vi "实时小时数据单参数上传.vi"(0 "参数数值":T1={"CODMn"=TRUE, "CODCr"=TRUE, "DO"=TRUE, "铜"=TRUE, "PH"=TRUE, "氨氮"=TRUE, "比电导率"=TRUE, "水温"=TRUE, "COD"=TRUE, "浊度"=TRUE, "总氮"=TRUE, "总磷"=TRUE, "叶绿素a"=TRUE, "藻密度"=TRUE, "水位"=TRUE, "流速"=TRUE, "瞬时流量"=TRUE, "累积流量"=TRUE, "亚硝氮"=TRUE, "硫化物"=TRUE, "ORP"=TRUE, "铅"=TRUE, "镉"=TRUE, "锌"=TRUE, "镍"=TRUE, "锰"=TRUE, "汞"=TRUE}) -> (4 "数据发送起始时间":timestamp format="%<%.3X\n%Y/%m/%d>T", 15 "error out":errorcluster)   [LabVIEW 2016, in "数据传输系统.lvlib"]
uses:
  <vilib>/Utility/config.llb/Write Key (String).vi
  <vilib>/Utility/config.llb/NI_LVConfig.lvlib
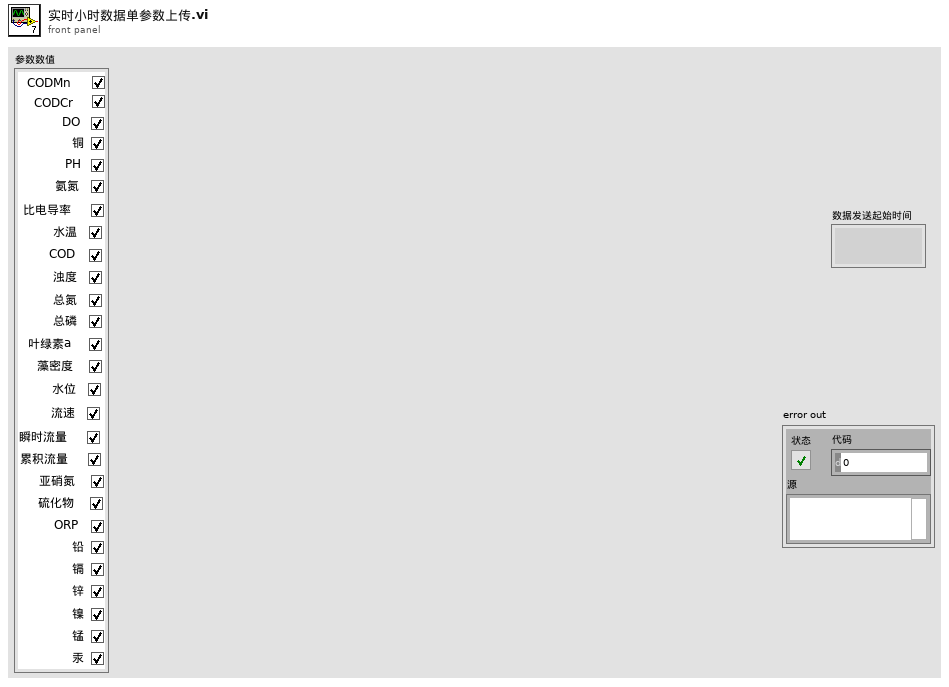
[diagram p1: front panel]
types:
  T1 = cluster{"CODMn":bool, "CODCr":bool, "DO":bool, "铜":bool, "PH":bool, "氨氮":bool, "比电导率":bool, "水温":bool, "COD":bool, "浊度":bool, "总氮":bool, "总磷":bool, "叶绿素a":bool, "藻密度":bool, "水位":bool, "流速":bool, "瞬时流量":bool, "累积流量":bool, "亚硝氮":bool, "硫化物":bool, "ORP":bool, "铅":bool, "镉":bool, "锌":bool, "镍":bool, "锰":bool, "汞":bool}
  T2 = cluster{"CODMn":bool, "CODCr":bool, "DO":bool, "铜":bool, "PH":bool, "氨氮":bool, "比电导率":bool, "水温":bool, "COD":bool, "浊度":bool, "总氮":bool, "总磷":bool, "叶绿素a":bool, "藻密度":bool, "水位":bool, "流速":bool, "瞬时流量":bool, "累积流量":bool, "亚硝酸盐":bool, "硫化物":bool, "ORP":bool, "铅":bool, "镉":bool, "锌":bool, "镍":bool, "锰":bool, "汞":bool}
  T3 = cluster{"time1":string, "time2":string, "time3":string, "time4":string, "time5":string, "time6":string, "time7":string, "time8":string, "time9":string, "time10":string, "time11":string, "time12":string, "time13":string, "time14":string, "time15":string, "time16":string, "time17":string, "time18":string, "time19":string, "time20":string, "time21":string, "time22":string, "time23":string, "time24":string, "time25":string, "time26":string, "time27":string}
  T4 = typedef "NI_LVConfig.lvlib/Config Data RefNum.ctl" = refnum<k1>
  T5 = cluster{"水样数据索引[0]":string, "水样数据索引[1]":string, "水样数据索引[2]":string, "水样数据索引[3]":string, "水样数据索引[4]":string, "水样数据索引[5]":string, "水样数据索引[6]":string, "水样数据索引[7]":string, "水样数据索引[8]":string, "水样数据索引[9]":string, "水样数据索引[10]":string, "水样数据索引[11]":string, "水样数据索引[12]":string, "水样数据索引[13]":string, "水样数据索引[14]":string, "水样数据索引[15]":string, "水样数据索引[16]":string, "水样数据索引[17]":string, "水样数据索引[18]":string, "水样数据索引[19]":string, "水样数据索引[20]":string, "水样数据索引[21]":string, "水样数据索引[22]":string, "水样数据索引[23]":string, "水样数据索引[24]":string, "水样数据索引[25]":string, "水样数据索引[26]":string}
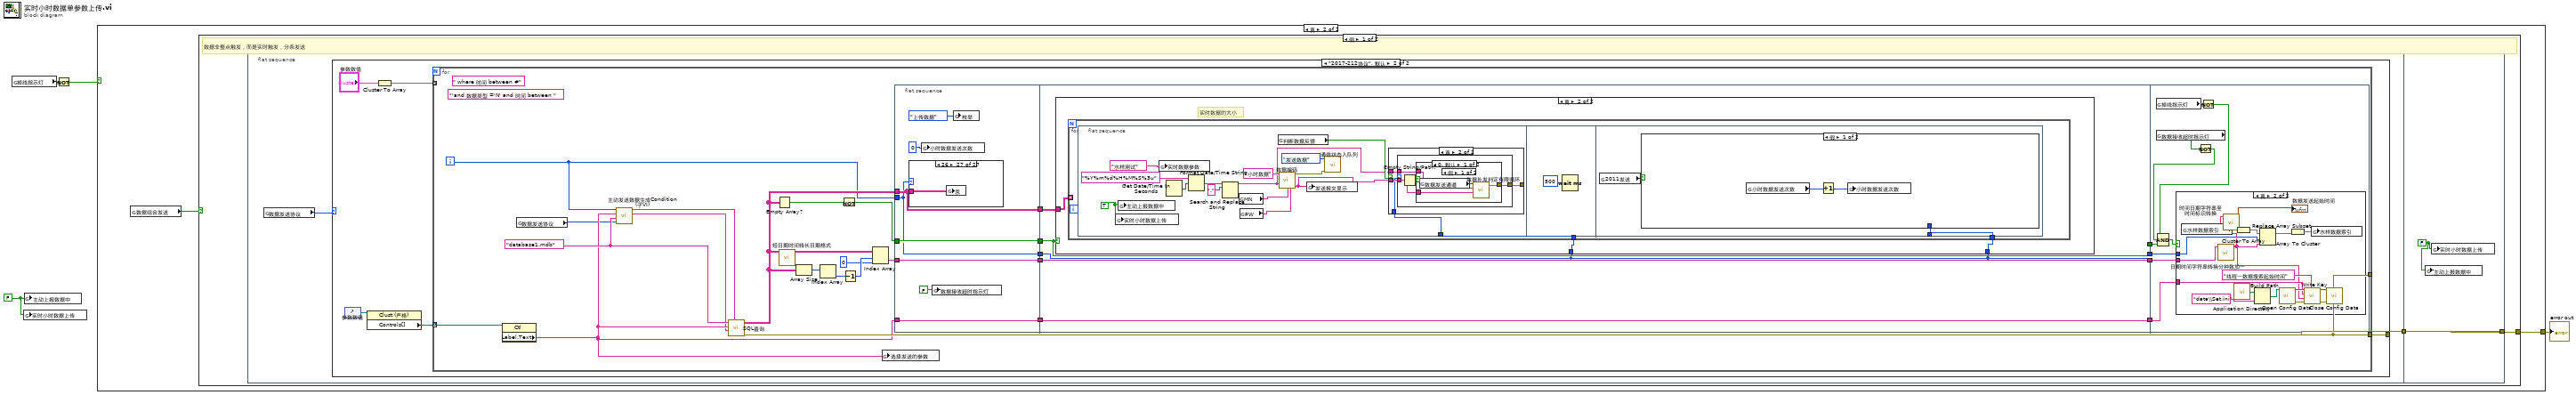
[diagram p0: block diagram]
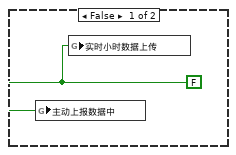
[diagram p2: hidden frame]
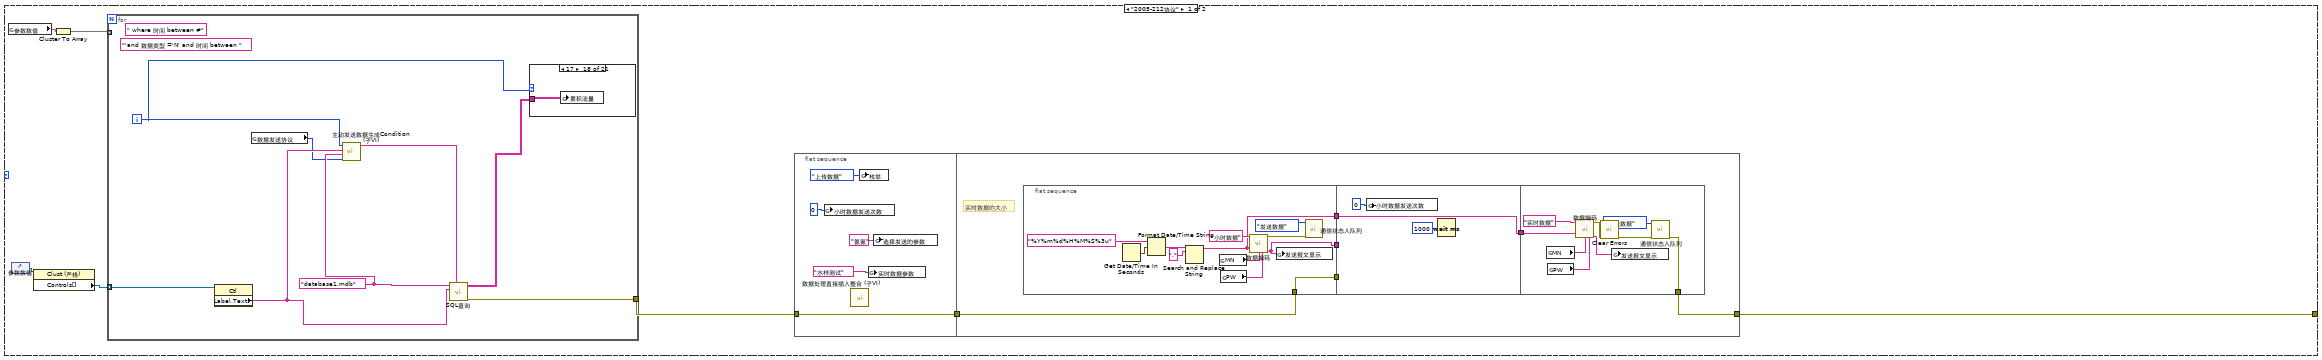
[diagram p3: hidden frame]
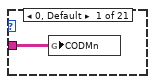
[diagram p4: hidden frame]
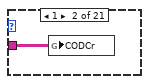
[diagram p5: hidden frame]
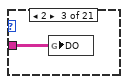
[diagram p6: hidden frame]
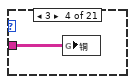
[diagram p7: hidden frame]
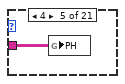
[diagram p8: hidden frame]
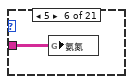
[diagram p9: hidden frame]
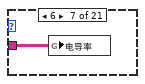
[diagram p10: hidden frame]
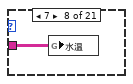
[diagram p11: hidden frame]
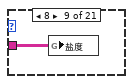
[diagram p12: hidden frame]
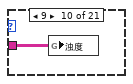
[diagram p13: hidden frame]
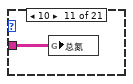
[diagram p14: hidden frame]
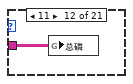
[diagram p15: hidden frame]
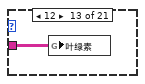
[diagram p16: hidden frame]
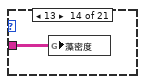
[diagram p17: hidden frame]
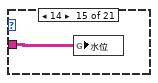
[diagram p18: hidden frame]
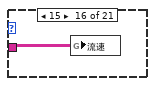
[diagram p19: hidden frame]
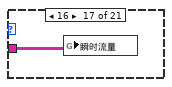
[diagram p20: hidden frame]
diagram:
  w1 = FALSE ("小时数据上传")
  n1 = global read "全局 数据发送重叠.vi" "掉线指示灯"() -> (w4:bool)
  n2 = global write "全局1.vi" "实时小时数据上传"(w1) -> ()
  n3 = global write "全局 数据发送重叠.vi" "主动上报数据中"(w1) -> ()
  n4 = Not(x=w4) -> (.not. x?=w3:bool)
  n5 = case shown="真" w3 {
    tunnel: [_ w7] -> w2
    frame False {
      w5 = FALSE ("小时数据上传")
      n6 = global write "全局 数据发送重叠.vi" "主动上报数据中"(w5) -> ()
      n7 = global write "全局1.vi" "实时小时数据上传"(w5) -> ()
    }
    frame True {
      n8 = global read "断电保存全局.vi" "数据组合发送"() -> (w6:bool)
      n9 = case shown="假" w6 {
        tunnel: [w8 _] -> w7
        frame False {
          # "数据非整点触发，而是实时触发，分条发送"
          n10 = flat-sequence {
            tunnel: [w11] -> w9
            tunnel: [w241] -> w8
            tunnel: w9 -> [w241]
            frame #0 {
              n11 = global read "断电保存全局.vi" "数据发送协议"() -> (w10:enum16{"2005-212协议", "2017-212协议"})
              n12 = case shown="\"2017-212协议\", 默认" w10 {
                tunnel: [w12 w86] -> w11
                frame "2005-212协议" {
                  n13 = global read "全局1.vi" "参数数值"() -> (w15:T2)
                  n14 = control-ref of="参数数值"() -> (w14:refnum<vi>)
                  n15 = property class="Clust (严格)"(reference=w14) -> ("Controls[]"=w13:refnum<vi>[])  [unwired: 1 in, 2 out]
                  n16 = Cluster To Array(cluster=w15) -> (array=w18:bool[])
                  n17 = for {
                    tunnel: w18 -> [_] mode=indexing
                    tunnel: [w61] -> w17
                    tunnel: w13 -> [w56] mode=indexing
                    i -> [w54]
                    (unwired) " where 时间 between #"
                    w59 = "database1.mdb" ("database")
                    (unwired) "'and 数据类型 ='N' and 时间 between "
                    n18 = property class="Ctl"(reference=w56) -> ("Label.Text"=w60:string)  [unwired: 1 in, 2 out]
                    n19 = global read "断电保存全局.vi" "数据发送协议"() -> (w57:enum16{"2005-212协议", "2017-212协议"})
                    n20 = call "主动发送数据生成Condition(子VI).vi"("数据发送协议"=w57, "database"=w59, "Label.Text"=w60, "数值"=w54) -> ("CONDITION"=w58:string)  [unwired: 6 in, 1 out]
                    n21 = call "SQL查询.vi"("condition"=w58, "table输入"=w60, "database"=w59) -> ("error out"=w61:errorcluster, "data"=w55:string[][])  [unwired: 6 in, 1 out]
                    n22 = case shown="17" w54 {
                      tunnel: w55 -> [w62 w63 w64 w65 w66 w67 w68 w69 w70 w71 w72 w73 w74 w75 w76 w77 w78 w79 w80 w81 w82]
                      frame 0, Default {
                        n23 = global write "全局 所有参数.vi" "CODMn"(w62) -> ()
                      }
                      frame 1 {
                        n24 = global write "全局 所有参数.vi" "CODCr"(w63) -> ()
                      }
                      frame 2 {
                        n25 = global write "全局 所有参数.vi" "DO"(w64) -> ()
                      }
                      frame 3 {
                        n26 = global write "全局 所有参数.vi" "铜"(w65) -> ()
                      }
                      frame 4 {
                        n27 = global write "全局 所有参数.vi" "PH"(w66) -> ()
                      }
                      frame 5 {
                        n28 = global write "全局 所有参数.vi" "氨氮"(w67) -> ()
                      }
                      frame 6 {
                        n29 = global write "全局 所有参数.vi" "电导率"(w68) -> ()
                      }
                      frame 7 {
                        n30 = global write "全局 所有参数.vi" "水温"(w69) -> ()
                      }
                      frame 8 {
                        n31 = global write "全局 所有参数.vi" "盐度"(w70) -> ()
                      }
                      frame 9 {
                        n32 = global write "全局 所有参数.vi" "浊度"(w71) -> ()
                      }
                      frame 10 {
                        n33 = global write "全局 所有参数.vi" "总氮"(w72) -> ()
                      }
                      frame 11 {
                        n34 = global write "全局 所有参数.vi" "总磷"(w73) -> ()
                      }
                      frame 12 {
                        n35 = global write "全局 所有参数.vi" "叶绿素"(w74) -> ()
                      }
                      frame 13 {
                        n36 = global write "全局 所有参数.vi" "藻密度"(w75) -> ()
                      }
                      frame 14 {
                        n37 = global write "全局 所有参数.vi" "水位"(w76) -> ()
                      }
                      frame 15 {
                        n38 = global write "全局 所有参数.vi" "流速"(w77) -> ()
                      }
                      frame 16 {
                        n39 = global write "全局 所有参数.vi" "瞬时流量"(w78) -> ()
                      }
                      frame 17 {
                        n40 = global write "全局 所有参数.vi" "累积流量"(w79) -> ()
                      }
                      frame 18 {
                        n41 = global write "全局 所有参数.vi" "亚硝酸盐"(w80) -> ()
                      }
                      frame 19 {
                        n42 = global write "全局 所有参数.vi" "硫化物"(w81) -> ()
                      }
                      frame 20 {
                        n43 = global write "全局 所有参数.vi" "ORP"(w82) -> ()
                      }
                    }
                  }
                  n44 = flat-sequence {
                    tunnel: w17 -> [w19]
                    tunnel: [w19] -> w16
                    tunnel: w16 -> [w27]
                    tunnel: [w26] -> w12
                    frame #0 {
                      n45 = global write "全局 小时数据发送次数.vi" "小时数据发送次数"(0 ("小时数据发送次数")) -> ()
                      n46 = call "数据处理直接插入整合 (子VI).vi"() -> ()  [unwired: 12 in]
                      n47 = global write "全局1.vi" "枚举"(enum16{"返回请求应答", "上传数据", "返回执行结果"}."上传数据" ("枚举")) -> ()
                      n48 = global write "全局 实时数据参数.vi" "实时数据参数"("水样测试" ("实时数据参数")) -> ()
                      n49 = global write "全局 水样时间.vi" "选择发送的参数"("氨氮" ("选择发送的参数")) -> ()
                    }
                    frame #1 {
                      # "实时数据的大小"
                      n50 = flat-sequence {
                        tunnel: [w36] -> w29
                        tunnel: [w31] -> w28
                        tunnel: w27 -> [w31]
                        tunnel: [w30] -> w25
                        tunnel: w29 -> [_]
                        tunnel: w28 -> [_]
                        tunnel: w25 -> [w42]
                        tunnel: [w42] -> w24
                        tunnel: [w47] -> w26
                        tunnel: w24 -> [w46]
                        frame #0 {
                          n51 = Get Date/Time In Seconds() -> (seconds since 1Jan1904=w39:timestamp)
                          n52 = Format Date/Time String(time format string (%c)="%Y%m%d%H%M%S%3u" ("时间格式字符串(%c)"), seconds (now)=w39) -> (date/time string=w40:string)  [unwired: 1 in]
                          n53 = Search and Replace String(input string=w40, search string="." ("搜索字符串")) -> (result string=w30:string)  [unwired: 6 in, 3 out]
                          n54 = global read "断电保存全局.vi" "MN"() -> (w34:string)
                          n55 = global read "断电保存全局.vi" "PW"() -> (w33:string)
                          n56 = call "数据编码.vi"("table输入"="小时数据" ("新元素/子数组"), "QN"=w30, "MN"=w34, "PW"=w33) -> ("错误常量"=w32:errorcluster, "通讯包字符串"=w36:string)  [unwired: 10 in]
                          n57 = global write "全局1.vi" "发送报文显示"(w36) -> ()
                          n58 = call "通信状态入队列.vi"("错误输入（无错误）"=w32, "枚举"=enum16{"打开连接", "发送数据", "读取数据", "数据处理", "关闭连接"}."发送数据") -> ()  [unwired: 9 in, 1 out]
                        }
                        frame #1 {
                          n59 = global write "全局 小时数据发送次数.vi" "小时数据发送次数"(0 ("小时数据发送次数")) -> ()
                          n60 = Wait (ms)(milliseconds to wait=u32 1000 ("等待时间（毫秒）")) -> ()  [unwired: 1 out]
                        }
                        frame #2 {
                          n61 = global read "断电保存全局.vi" "MN"() -> (w49:string)
                          n62 = global read "断电保存全局.vi" "PW"() -> (w50:string)
                          n63 = call "数据编码.vi"("table输入"="实时数据" ("新元素/子数组"), "QN"=w46, "MN"=w49, "PW"=w50) -> ("错误常量"=w48:errorcluster, "通讯包字符串"=w52:string)  [unwired: 10 in]
                          n64 = call <vilib>:"Clear Errors.vi"("error in (no error)"=w48) -> ("error out"=w45:errorcluster)  [unwired: 5 in, 1 out]
                          n65 = global write "全局1.vi" "发送报文显示"(w52) -> ()
                          n66 = call "通信状态入队列.vi"("错误输入（无错误）"=w45, "枚举"=enum16{"打开连接", "发送数据", "读取数据", "数据处理", "关闭连接"}."发送数据") -> ("错误输出"=w47:errorcluster)  [unwired: 9 in]
                        }
                      }
                    }
                  }
                }
                frame "2017-212协议", Default {
                  n67 = control-ref of="参数数值"() -> (w85:refnum<vi>)
                  n68 = property class="Clust (严格)"(reference=w85) -> ("Controls[]"=w84:refnum<vi>[])  [unwired: 1 in, 2 out]
                  n69 = Cluster To Array(cluster="参数数值") -> (array=w87:bool[])
                  n70 = for {
                    tunnel: w87 -> [_] mode=indexing
                    tunnel: [w99] -> w86
                    tunnel: [w99] -> _
                    tunnel: w84 -> [w89] mode=indexing
                    i -> [w90]
                    (unwired) " where 时间 between #"
                    w98 = "database1.mdb" ("database")
                    (unwired) "'and 数据类型 ='N' and 时间 between "
                    n71 = property class="Ctl"(reference=w89) -> ("Label.Text"=w97:string)  [unwired: 1 in, 2 out]
                    n72 = global read "断电保存全局.vi" "数据发送协议"() -> (w96:enum16{"2005-212协议", "2017-212协议"})
                    n73 = call "主动发送数据生成Condition(子VI).vi"("数据发送协议"=w96, "database"=w98, "Label.Text"=w97, "数值"=w90) -> ("columns"=w88:string[], "CONDITION"=w113:string)  [unwired: 6 in]
                    n74 = call "SQL查询.vi"("condition"=w113, "columns"=w88, "table输入"=w97, "database"=w98) -> ("error out"=w99:errorcluster, "data"=w93:string[][])  [unwired: 5 in, 1 out]
                    n75 = Empty Array?(array=w93) -> (empty?=w112:bool)
                    n76 = call "短日期时间转长日期格式.vi"("data"=w93) -> ("输出数组"=w111:string[][])  [unwired: 10 in]
                    n77 = Array Size(array=w93) -> (size(s)=w95:i32[])
                    n78 = Index Array(array=w95) -> (element=w94:i32)  [unwired: 1 in]
                    n79 = Not(x=w112) -> (.not. x?=w108:bool)
                    n80 = Decrement(x=w94) -> (x-1=w92:i32)
                    n81 = Index Array(array=w111, index (row)=w92, index (col)=0 ("禁用的索引 (列)")) -> (element=w105:string)
                    n82 = global write "全局 水样时间.vi" "选择发送的参数"(w97) -> ()
                    n83 = flat-sequence {
                      tunnel: [w121] -> w110
                      tunnel: [w120] -> w109
                      tunnel: w108 -> [w121]
                      tunnel: w93 -> [w120]
                      tunnel: w90 -> [w115]
                      tunnel: w97 -> [w117]
                      tunnel: [w117] -> w106
                      tunnel: w105 -> [w116]
                      tunnel: [w116] -> w103
                      tunnel: [w115] -> w100
                      tunnel: w110 -> [w150]
                      tunnel: w109 -> [w153]
                      tunnel: [w152] -> w107
                      tunnel: w106 -> [w152]
                      tunnel: [w151] -> w104
                      tunnel: w103 -> [w151]
                      tunnel: [w150] -> w102
                      tunnel: [w149] -> w101
                      tunnel: w100 -> [w149]
                      tunnel: w107 -> [w222]
                      tunnel: w104 -> [w221]
                      tunnel: w102 -> [w219]
                      tunnel: w101 -> [w220]
                      frame #0 {
                        n84 = case shown="26" w115 {
                          tunnel: w120 -> [w122 w123 w124 w125 w126 w127 w128 w129 w130 w131 w132 w133 w134 w135 w136 w137 w138 w139 w140 w141 w142 w143 w144 w145 w146 w147 w148]
                          frame 0, Default {
                            n85 = global write "全局 所有参数.vi" "CODMn"(w122) -> ()
                          }
                          frame 1 {
                            n86 = global write "全局 所有参数.vi" "CODCr"(w123) -> ()
                          }
                          frame 2 {
                            n87 = global write "全局 所有参数.vi" "DO"(w124) -> ()
                          }
                          frame 3 {
                            n88 = global write "全局 所有参数.vi" "铜"(w125) -> ()
                          }
                          frame 4 {
                            n89 = global write "全局 所有参数.vi" "PH"(w126) -> ()
                          }
                          frame 5 {
                            n90 = global write "全局 所有参数.vi" "氨氮"(w127) -> ()
                          }
                          frame 6 {
                            n91 = global write "全局 所有参数.vi" "电导率"(w128) -> ()
                          }
                          frame 7 {
                            n92 = global write "全局 所有参数.vi" "水温"(w129) -> ()
                          }
                          frame 8 {
                            n93 = global write "全局 所有参数.vi" "盐度"(w130) -> ()
                          }
                          frame 9 {
                            n94 = global write "全局 所有参数.vi" "浊度"(w131) -> ()
                          }
                          frame 10 {
                            n95 = global write "全局 所有参数.vi" "总氮"(w132) -> ()
                          }
                          frame 11 {
                            n96 = global write "全局 所有参数.vi" "总磷"(w133) -> ()
                          }
                          frame 12 {
                            n97 = global write "全局 所有参数.vi" "叶绿素"(w134) -> ()
                          }
                          frame 13 {
                            n98 = global write "全局 所有参数.vi" "藻密度"(w135) -> ()
                          }
                          frame 14 {
                            n99 = global write "全局 所有参数.vi" "水位"(w136) -> ()
                          }
                          frame 15 {
                            n100 = global write "全局 所有参数.vi" "流速"(w137) -> ()
                          }
                          frame 16 {
                            n101 = global write "全局 所有参数.vi" "瞬时流量"(w138) -> ()
                          }
                          frame 17 {
                            n102 = global write "全局 所有参数.vi" "累积流量"(w139) -> ()
                          }
                          frame 18 {
                            n103 = global write "全局 所有参数.vi" "亚硝酸盐"(w140) -> ()
                          }
                          frame 19 {
                            n104 = global write "全局 所有参数.vi" "硫化物"(w141) -> ()
                          }
                          frame 20 {
                            n105 = global write "全局 所有参数.vi" "ORP"(w142) -> ()
                          }
                          frame 21 {
                            n106 = global write "全局 所有参数.vi" "铅"(w143) -> ()
                          }
                          frame 22 {
                            n107 = global write "全局 所有参数.vi" "镉"(w144) -> ()
                          }
                          frame 23 {
                            n108 = global write "全局 所有参数.vi" "锌"(w145) -> ()
                          }
                          frame 24 {
                            n109 = global write "全局 所有参数.vi" "镍"(w146) -> ()
                          }
                          frame 25 {
                            n110 = global write "全局 所有参数.vi" "锰"(w147) -> ()
                          }
                          frame 26 {
                            n111 = global write "全局 所有参数.vi" "汞"(w148) -> ()
                          }
                        }
                        n112 = global write "全局 小时数据发送次数.vi" "小时数据发送次数"(0 ("小时数据发送次数")) -> ()
                        n113 = global write "全局 数据发送重叠.vi" "数据接收超时指示灯"(FALSE ("数据接收超时指示灯")) -> ()
                        n114 = global write "全局1.vi" "枚举"(enum16{"返回请求应答", "上传数据", "返回执行结果"}."上传数据" ("枚举")) -> ()
                      }
                      frame #1 {
                        n115 = case shown="真" w150 {
                          tunnel: w153 -> [_ w156]
                          tunnel: w149 -> [_ w155]
                          tunnel: w149 -> [_ w154]
                          frame False {
                          }
                          frame True {
                            # "实时数据的大小"
                            n116 = for {
                              tunnel: w156 -> [_] mode=indexing
                              tunnel: w155 -> [w158]
                              tunnel: w154 -> [w157]
                              n117 = flat-sequence {
                                tunnel: w158 -> [w173]
                                tunnel: w157 -> [w187]
                                frame #0 {
                                w160 = TRUE ("小时数据上传")
                                n118 = global write "全局1.vi" "实时小时数据上传"(w160) -> ()
                                n119 = global write "全局 数据发送重叠.vi" "主动上报数据中"(w160) -> ()
                                n120 = global write "全局 实时数据参数.vi" "实时数据参数"("水样测试" ("实时数据参数")) -> ()
                                n121 = Get Date/Time In Seconds() -> (seconds since 1Jan1904=w170:timestamp)
                                n122 = Format Date/Time String(time format string (%c)="%Y%m%d%H%M%S%3u" ("时间格式字符串(%c)"), seconds (now)=w170) -> (date/time string=w171:string)  [unwired: 1 in]
                                n123 = Search and Replace String(input string=w171, search string="." ("搜索字符串")) -> (result string=w159:string)  [unwired: 6 in, 3 out]
                                n124 = global read "断电保存全局.vi" "MN"() -> (w166:string)
                                n125 = global read "断电保存全局.vi" "PW"() -> (w165:string)
                                n126 = global read "断电保存全局.vi" "判断数据反馈"() -> (w162:bool)
                                n127 = call "数据编码.vi"("table输入"="小时数据" ("新元素/子数组"), "QN"=w159, "MN"=w166, "PW"=w165) -> ("错误常量"=w163:errorcluster, "通讯包字符串"=w161:string)  [unwired: 10 in]
                                n128 = global write "全局1.vi" "发送报文显示"(w161) -> ()
                                n129 = call "通信状态入队列.vi"("错误输入（无错误）"=w163, "枚举"=enum16{"打开连接", "发送数据", "读取数据", "数据处理", "关闭连接"}."发送数据") -> ()  [unwired: 9 in, 1 out]
                                n130 = case shown="真" w162 {
                                tunnel: [_ w177] -> _
                                tunnel: w161 -> [_ w176]
                                tunnel: w173 -> [_ w175]
                                tunnel: w159 -> [_ w174]
                                frame False {
                                }
                                frame True {
                                n131 = case shown="0, 默认" w175 {
                                tunnel: [w180 _] -> w177
                                tunnel: w176 -> [w179 _]
                                tunnel: w174 -> [w178 _]
                                frame 0, Default {
                                n132 = Empty String/Path?(string/path=w179) -> (empty?=w181:bool)
                                n133 = case shown="假" w181 {
                                tunnel: [w185 _] -> w180
                                tunnel: w179 -> [w184 _]
                                tunnel: w178 -> [w182 _]
                                frame False {
                                n134 = global read "断电保存全局.vi" "数据发送通道"() -> (w183:enum16{"TCP", "VISA"})
                                n135 = call "数据补发判定有限循环.vi"("数据输入"=w184, "QN"=w182, "数据发送通道"=w183) -> ("error out"=w185:errorcluster)  [unwired: 8 in]
                                }
                                frame True {
                                }
                                }
                                }
                                frame 14..17 {
                                }
                                }
                                }
                                }
                                }
                                frame #1 {
                                n136 = Wait (ms)(milliseconds to wait=u32 500 ("等待时间（毫秒）")) -> ()  [unwired: 1 out]
                                }
                                frame #2 {
                                n137 = global read "断电保存全局.vi" "2011发送"() -> (w188:bool)
                                n138 = case shown="假" w188 {
                                tunnel: w187 -> [_ w205]
                                frame False {
                                n139 = global read "全局 小时数据发送次数.vi" "小时数据发送次数"() -> (w190:i32)
                                n140 = Increment(x=w190) -> (x+1=w189:i32)
                                n141 = global write "全局 小时数据发送次数.vi" "小时数据发送次数"(w189) -> ()
                                }
                                frame True {
                                n142 = Get Date/Time In Seconds() -> (seconds since 1Jan1904=w193:timestamp)
                                n143 = Format Date/Time String(time format string (%c)="%Y%m%d%H%M%S%3u" ("时间格式字符串(%c)"), seconds (now)=w193) -> (date/time string=w194:string)  [unwired: 1 in]
                                n144 = global read "断电保存全局.vi" "MN"() -> (w200:string)
                                n145 = global read "断电保存全局.vi" "PW"() -> (w199:string)
                                n146 = Search and Replace String(input string=w194, search string="." ("搜索字符串")) -> (result string=w191:string)  [unwired: 6 in, 3 out]
                                n147 = global write "全局 实时数据参数.vi" "实时数据参数"("水样测试" ("实时数据参数")) -> ()
                                n148 = call "数据编码.vi"("table输入"="实时数据" ("新元素/子数组"), "QN"=w191, "MN"=w200, "PW"=w199) -> ("错误常量"=w201:errorcluster, "通讯包字符串"=w196:string)  [unwired: 10 in]
                                n149 = global write "全局1.vi" "发送报文显示"(w196) -> ()
                                n150 = call "通信状态入队列.vi"("错误输入（无错误）"=w201, "枚举"=enum16{"打开连接", "发送数据", "读取数据", "数据处理", "关闭连接"}."发送数据") -> ("错误输出"=w198:errorcluster)  [unwired: 9 in]
                                n151 = global read "断电保存全局.vi" "判断数据反馈"() -> (w197:bool)
                                n152 = case shown="真" w197 {
                                tunnel: w196 -> [_ w209]
                                tunnel: w198 -> [_ w208]
                                tunnel: w205 -> [_ w207]
                                tunnel: w191 -> [_ w206]
                                frame False {
                                }
                                frame True {
                                n153 = case shown="0, 默认" w207 {
                                tunnel: w209 -> [w213 _]
                                tunnel: w208 -> [w212 _]
                                tunnel: w206 -> [w210 _]
                                frame 0, Default {
                                n154 = global read "断电保存全局.vi" "数据发送通道"() -> (w211:enum16{"TCP", "VISA"})
                                n155 = call "数据补发判定有限循环.vi"("错误输入（无错误）"=w212, "数据输入"=w213, "QN"=w210, "数据发送通道"=w211) -> ()  [unwired: 7 in, 1 out]
                                }
                                frame 14..17 {
                                }
                                }
                                }
                                }
                                }
                                }
                                }
                              }
                            }
                          }
                        }
                      }
                      frame #2 {
                        n156 = global read "全局 数据发送重叠.vi" "掉线指示灯"() -> (w215:bool)
                        n157 = global read "全局 数据发送重叠.vi" "数据接收超时指示灯"() -> (w216:bool)
                        n158 = Not(x=w216) -> (.not. x?=w217:bool)
                        n159 = Not(x=w215) -> (.not. x?=w214:bool)
                        n160 = Compound Arithmetic op=AND ("复合运算")(w214, w217, w219) -> (w218:bool)
                        n161 = case shown="真" w218 {
                          tunnel: w221 -> [_ w230]
                          tunnel: w220 -> [_ w224]
                          tunnel: w222 -> [_ w231]
                          frame False {
                          }
                          frame True {
                            n162 = global read "全局 水样时间.vi" "水样数据索引"() -> (w225:T3)
                            n163 = call "日期时间字符串转换分钟数加一.vi"("data[0]"=w230) -> ("日期/时间字符串"=w223:string)  [unwired: 10 in]
                            n164 = call "时间日期字符串至时间标识转换.vi"("时间日期字符串"=w223) -> ("时间标识"=→"数据发送起始时间":timestamp)  [unwired: 10 in]
                            n165 = call <vilib>:"Application Directory.vi"() -> ("Application Directory"=w232:path)
                            n166 = Cluster To Array(cluster=w225) -> (array=w226:string[])
                            n167 = Build Path(base path=w232, name or relative path="data\\Set.ini" ("名称或相对路径")) -> (appended path=w234:path)
                            n168 = Replace Array Subset(array=w226, new element=w223, index=w224) -> (w227:string[])
                            n169 = call <vilib>:"Open Config Data.vi"("configuration file path"=w234) -> ("error out"=w236:errorcluster, "refnum"=w235:T4)  [unwired: 8 in, 1 out]
                            n170 = Array To Cluster(array=w227) -> (cluster=w228:T5)
                            n171 = call-poly <vilib>:"Write Key.vi"("section"="线程一数据搜索起始时间", "error in (no error)"=w236, "value"=w223, "key"=w231, "refnum"=w235) -> ("error out"=w238:errorcluster, "refnum out"=w237:T4)  [unwired: 4 in, 1 out]
                            n172 = global write "全局 水样时间.vi" "水样数据索引"(w228) -> ()
                            n173 = call <vilib>:"Close Config Data.vi"("error in (no error)"=w238, "refnum"=w237) -> ()  [unwired: 8 in, 2 out]
                          }
                        }
                      }
                    }
                  }
                }
              }
            }
            frame #1 {
              w240 = FALSE ("小时数据上传")
              n174 = global write "全局 数据发送重叠.vi" "主动上报数据中"(w240) -> ()
              n175 = global write "全局1.vi" "实时小时数据上传"(w240) -> ()
            }
          }
        }
        frame True {
          # "数据整点触发，整条发送"
          n176 = flat-sequence {
            frame #0 {
              n177 = global read "断电保存全局.vi" "数据发送通道"() -> (w242:enum16{"TCP", "VISA"})
              n178 = global read "断电保存全局.vi" "MN"() -> (w244:string)
              n179 = global read "断电保存全局.vi" "PW"() -> (w243:string)
              n180 = call "数据全参数一起发送整点触发.vi"("数据发送通道"=w242, "PW"=w243, "MN"=w244) -> ()  [unwired: 8 in]
            }
            frame #1 {
              w245 = FALSE ("主动上报数据中")
              n181 = global write "全局 数据发送重叠.vi" "主动上报数据中"(w245) -> ()
              n182 = global write "全局1.vi" "实时小时数据上传"(w245) -> ()
            }
          }
        }
      }
    }
  }
  "error out" <- w2
